vi "Open Reference to SubVI.vi"(8 "error in (no error)":errorcluster, 10 "SubVI Name":string, 11 "VI in":refnum<vi>) -> (0 "error out":errorcluster, 2 "SubVI Refnum":refnum<vi>, 3 "VI out":refnum<vi>)   [LabVIEW 2020, in "Responsive Mock Class Generator.lvclass"]
uses:
  Responsive Mock Class Generator.lvclass
  <vilib>/Utility/traverseref.llb/TRef TravTarget.ctl
  <vilib>/Utility/traverseref.llb/VI Scripting - Traverse.lvlib
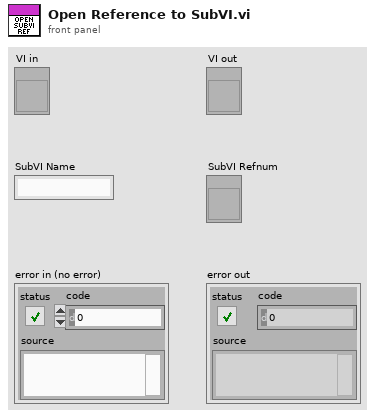
[diagram p1: front panel]
types:
  T1 = typedef "TRef TravTarget.ctl" = enum16{"FP", "BD", "Other"}
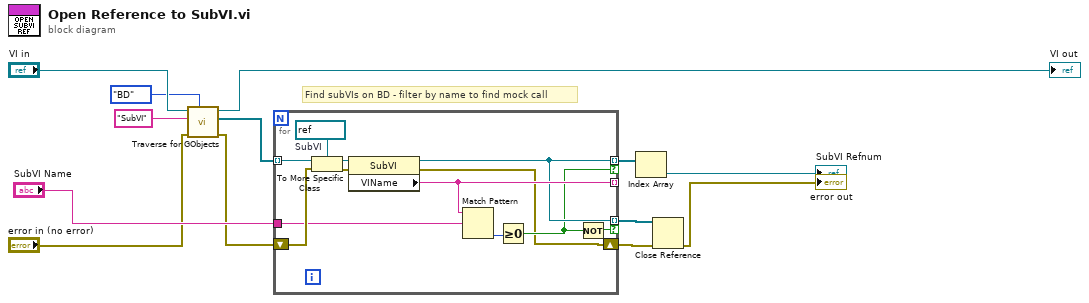
[diagram p0: block diagram]
diagram:
  # "Find subVIs on BD - filter by name to find mock call"
  n1 = call <vilib>:"Traverse for GObjects.vi"("Traverse Target"=TRef_TravTarget."BD", "error in (no error)"="error in (no error)", "Class Name"="SubVI", "VI Refnum"="VI in") -> ("error out"=w3:errorcluster, "References"=w2:refnum<vi>[], "dup VI Refnum"=→"VI out":refnum<vi>)  [unwired: 4 in, 1 out]
  n2 = for {
    tunnel: w2 -> [w25] mode=indexing
    tunnel: [w18] -> w8 mode=indexing if=w17
    tunnel: [w20] -> _ mode=indexing
    tunnel: [w18] -> w5 mode=indexing if=w16
    shift-right: [w15] -> w6
    shift-left: w3 -> [w21]
    tunnel: "SubVI Name" -> [w14]
    w23 = refnum<vi> refnum  # SubVI
    n3 = To More Specific Class(target class=w23, reference=w25, error in=w21) -> (specific class reference=w24:refnum<vi>, error out=w22:errorcluster)
    n4 = property class="SubVI"(reference=w24, error in=w22) -> (reference out=w18:refnum<vi>, error out=w15:errorcluster, "VIName"=w20:string)
    n5 = Match Pattern(string=w20, regular expression=w14) -> (offset past match=w19:i32)  [unwired: 1 in, 3 out]
    n6 = Greater Or Equal To 0?(x=w19) -> (x >= 0?=w17:bool)
    n7 = Not(x=w17) -> (.not. x?=w16:bool)
  }
  n8 = Index Array(array=w8) -> (element=→"SubVI Refnum":refnum<vi>)  [unwired: 1 in]
  n9 = Close Reference(reference=w5, error in (no error)=w6) -> (error out=→"error out":errorcluster)
